vi "Set Target Time.vi"() -> ()   [LabVIEW 2021]
uses:
  <vilib>/nisyscfg/nisyscfg.lvlib
panel:
  out "Incomplete":string[](array[string])
  out "Completed":string[](array[string])
  out "Detected Systems":string[](array[string])
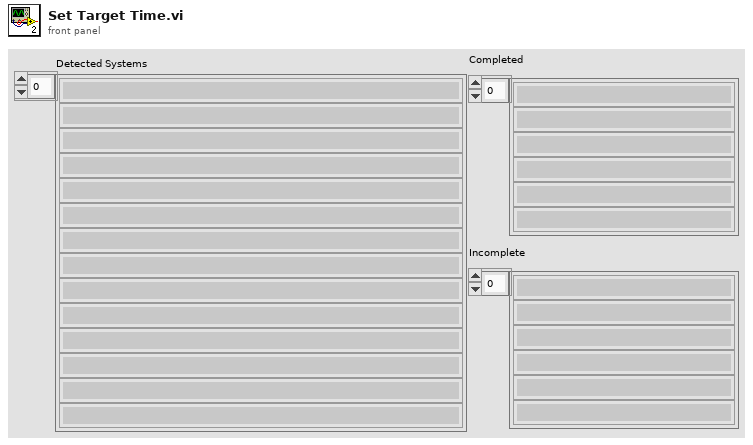
[diagram p1: front panel]
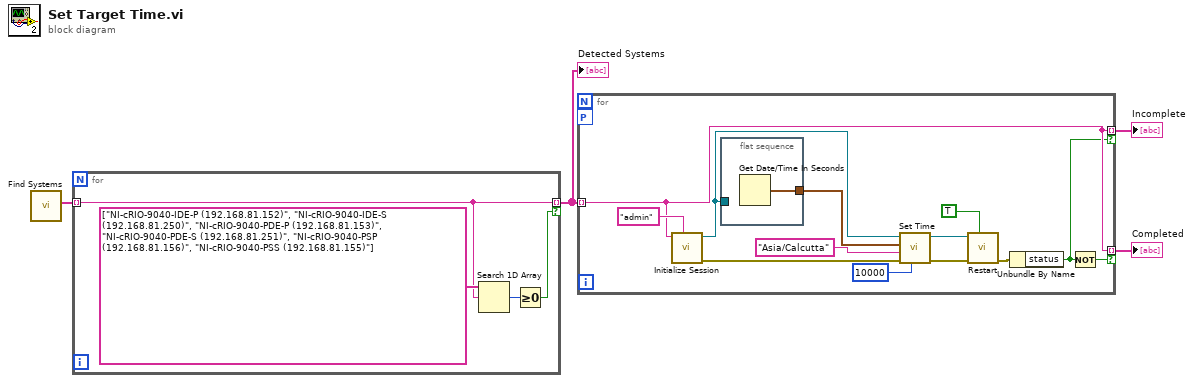
[diagram p0: block diagram]
diagram:
  n1 = call <vilib>:"Find Systems.vi"() -> ("Detected Systems"=w4:string[])  [unwired: 9 in, 2 out]
  n2 = for {
    tunnel: w4 -> [w7] mode=indexing
    tunnel: [w7] -> w3 mode=indexing if=w5
    n3 = Search 1D Array(1D array=string[] ["NI-cRIO-9040-IDE-P (192.168.81.152)", "NI-cRIO-9040-IDE-S (192.168.81.250)", "NI-cRIO-9040-PDE-P (192.168.81.153)", "NI-cRIO-9040-PDE-S (192.168.81.251)", "NI-cRIO-9040-PSP (192.168.81.156)", "NI-cRIO-9040-PSS (192.168.81.155)"] ("Detected Systems 2"), element=w7) -> (index of element=w6:i32)  [unwired: 1 in]
    n4 = Greater Or Equal To 0?(x=w6) -> (x >= 0?=w5:bool)
  }
  "Detected Systems" <- w3
  n5 = for {
    tunnel: w3 -> [w11] mode=indexing
    workers-P: _ -> [_]
    tunnel: [w11] -> w2 mode=indexing if=w12
    tunnel: [w11] -> w1 mode=indexing if=w10
    n6 = call <vilib>:"Initialize Session.vi"("User Name"="admin", "Target (localhost)"=w11) -> ("error out"=w15:errorcluster, "Session out"=w9:refnum<k21>)  [unwired: 8 in]
    n7 = flat-sequence {
      tunnel: [w22] -> w20
      tunnel: w9 -> [_]
      frame #0 {
        n8 = Get Date/Time In Seconds() -> (seconds since 1Jan1904=w22:timestamp)
      }
    }
    n9 = call <vilib>:"Set Time.vi"("Remote Timeout (300,000 ms)"=u32 10000, "error in (no error)"=w15, "Time Zone"="Asia/Calcutta", "Time"=w20, "Session in (localhost)"=w9) -> ("error out"=w17:errorcluster, "Session out"=w19:refnum<k21>)  [unwired: 3 in, 2 out]
    n10 = call <vilib>:"Restart.vi"("Wait Until Complete (T)"=TRUE, "error in (no error)"=w17, "Session in"=w19) -> ("error out"=w13:errorcluster)  [unwired: 6 in, 2 out]
    n11 = Unbundle By Name(w13) -> ("status"=w10:bool)
    n12 = Not(x=w10) -> (.not. x?=w12:bool)
  }
  "Completed" <- w2
  "Incomplete" <- w1
